vi "getFileContent.vi"(2 "error in":errorcluster, 3 "file path":path) -> (0 "error out":errorcluster, 1 "byte array":u8[](array[numeric]))   [LabVIEW 2014]
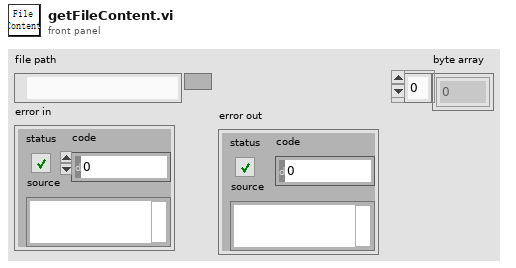
[diagram p1: front panel]
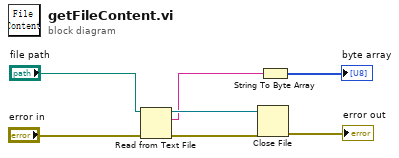
[diagram p0: block diagram]
diagram:
  n1 = Read from Text File(file (use dialog)="file path", error in="error in") -> (refnum out=w6:refnum<file>, text=w2:string, error out=w5:errorcluster)  [unwired: 2 in, 1 out]
  n2 = Close File(refnum=w6, error in=w5) -> (error out=→"error out":errorcluster)  [unwired: 1 out]
  n3 = String To Byte Array(string=w2) -> (unsigned byte array=→"byte array":u8[])
